vi "Get Surface Normal.vi"(9 "Triangle Index Array":u32[](array[numeric]), 11 "Vertex Array":cluster{"X":sgl, "Y":sgl, "Z":sgl}[](array[cluster])) -> (3 "Normal Array":cluster{"X":sgl, "Y":sgl, "Z":sgl}[](array[cluster]))   [LabVIEW 2020, in "3D Plot Datatype.lvclass"]
uses:
  <vilib>/Math Plots/3D Math Plots/3D Plot/3D Plot Datatype/3D Plot Datatype.lvclass
  <vilib>/Math Plots/3D Math Plots/3D Plot/3D Plot/3D Plot.lvclass
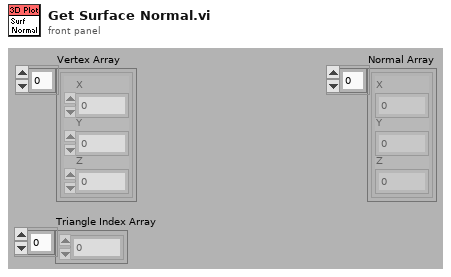
[diagram p1: front panel]
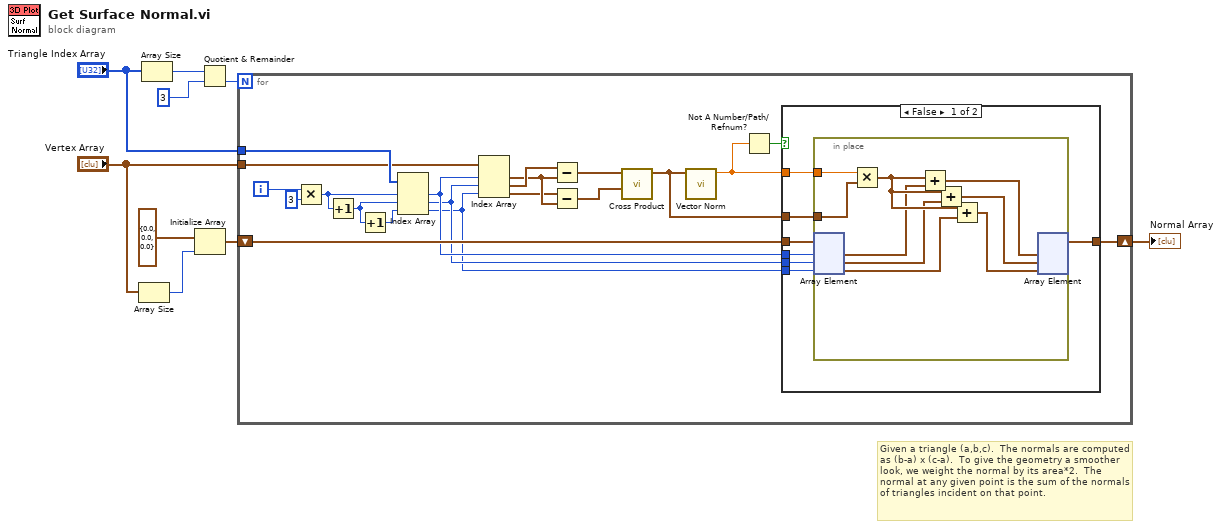
[diagram p0: block diagram]
diagram:
  # "Given a triangle (a,b,c).  The normals are computed as (b-a) x (c-a).  To give the geometry a smoother look, we weight the normal by its area*2.  The normal at any given point is the sum of the normals of triangles incident on that point."
  n1 = Array Size(array="Vertex Array") -> (size(s)=w7:i32)
  n2 = Array Size(array="Triangle Index Array") -> (size(s)=w3:i32)
  n3 = Initialize Array(cluster{"X":sgl, "Y":sgl, "Z":sgl} {"X"=0.0, "Y"=0.0, "Z"=0.0} ("3D Point"), w7) -> (w6:cluster{"X":sgl, "Y":sgl, "Z":sgl}[])
  n4 = Quotient & Remainder(x=w3, y=3) -> (floor(x/y)=w4:i32)  [unwired: 1 out]
  n5 = for {
    N: w4 -> [_]
    shift-right: [w12] -> w9
    shift-left: w6 -> [w16]
    tunnel: "Triangle Index Array" -> [w27]
    tunnel: "Vertex Array" -> [w23]
    i -> [w29]
    n6 = Multiply(x=w29, y=3) -> (x*y=w26:i32)
    n7 = Increment(x=w26) -> (x+1=w24:i32)
    n8 = Increment(x=w24) -> (x+1=w25:i32)
    n9 = Index Array(array=w27, index #1=w26, index #2=w24, index #3=w25) -> (element #1=w15:u32, element #2=w14:u32, element #3=w13:u32)
    n10 = Index Array(array=w23, index #1=w15, index #2=w14, index #3=w13) -> (element #1=w21:cluster{"X":sgl, "Y":sgl, "Z":sgl}, element #2=w22:cluster{"X":sgl, "Y":sgl, "Z":sgl}, element #3=w20:cluster{"X":sgl, "Y":sgl, "Z":sgl})
    n11 = Subtract(x=w22, y=w21) -> (x-y=w19:cluster{"X":sgl, "Y":sgl, "Z":sgl})
    n12 = Subtract(x=w20, y=w21) -> (x-y=w18:cluster{"X":sgl, "Y":sgl, "Z":sgl})
    n13 = call <vilib>:"Cross Product.vi"("Vector 2"=w18, "Vector 1"=w19) -> ("Vector Out"=w17:cluster{"X":sgl, "Y":sgl, "Z":sgl})  [unwired: 9 out]
    n14 = call <vilib>:"Vector Norm.vi"("Vector"=w17) -> ("Norm"=w11:sgl)  [unwired: 10 out]
    n15 = Not A Number/Path/Refnum?(number/path/refnum=w11) -> (NaN/Path/Refnum?=w10:bool)
    n16 = case shown="False" w10 {
      tunnel: w11 -> [w36 _]
      tunnel: w17 -> [w35 _]
      tunnel: w16 -> [w34 w46]
      tunnel: w15 -> [w33 _]
      tunnel: w14 -> [w32 _]
      tunnel: w13 -> [w31 _]
      tunnel: [w30 w46] -> w12
      frame False {
        n17 = in-place {
          in-place-border: w36 -> [w44]
          in-place-border: w35 -> [w43]
          n18 = in-place-array #1(w34, w33, w32, w31) -> (w42:cluster{"X":sgl, "Y":sgl, "Z":sgl}, w41:cluster{"X":sgl, "Y":sgl, "Z":sgl}, w40:cluster{"X":sgl, "Y":sgl, "Z":sgl})
          n19 = Multiply(x=w44, y=w43) -> (x*y=w45:cluster{"X":sgl, "Y":sgl, "Z":sgl})
          n20 = Add(x=w45, y=w42) -> (x+y=w39:cluster{"X":sgl, "Y":sgl, "Z":sgl})
          n21 = Add(x=w45, y=w41) -> (x+y=w38:cluster{"X":sgl, "Y":sgl, "Z":sgl})
          n22 = Add(x=w45, y=w40) -> (x+y=w37:cluster{"X":sgl, "Y":sgl, "Z":sgl})
          n23 = in-place-array #1(w39, w38, w37) -> (w30:cluster{"X":sgl, "Y":sgl, "Z":sgl}[])  [unwired: 3 out]
        }
      }
      frame True {
      }
    }
  }
  "Normal Array" <- w9
